vi "SH_readParams.vi"(8 "error in (no error)":errorcluster, 11 "ShapeletClass in":refnum<class "Shapelets Search Brute Force.lvclass">) -> (0 "error out":errorcluster, 1 "FeatureVectorLength":i32, 2 "NumberOfTrials":i32, 3 "ShapeletClass out":refnum<class "Shapelets Search Brute Force.lvclass">)   [LabVIEW 2016, in "Shapelets Search (Brute Force).lvlib" / "Shapelets Search Brute Force.lvclass"]
uses:
  Shapelets Search Brute Force.lvclass
  Shapelets Search Brute Force.lvclass/Shapelets Search Brute Force.ctl
panel:
  # "This VI is a part of BCI Design library, http://www.ru-bci.org \nCopyright © 2020, Sotnikov Peter, All rights reserved. License: CC BY-NC 4.0"
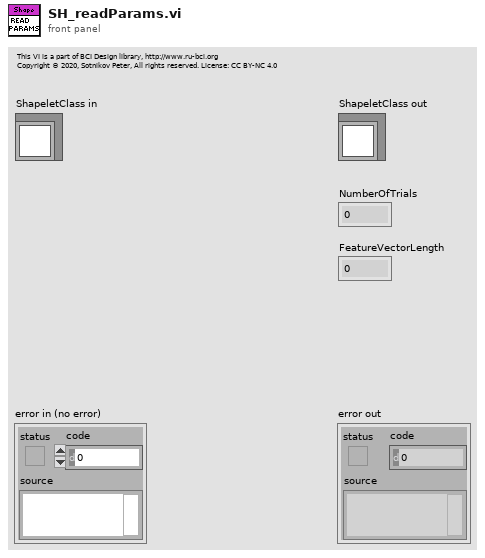
[diagram p1: front panel]
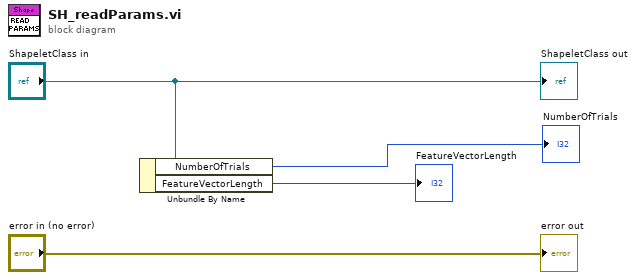
[diagram p0: block diagram]
diagram:
  n1 = Unbundle By Name("ShapeletClass in") -> ("NumberOfTrials"=→"NumberOfTrials":i32, "FeatureVectorLength"=→"FeatureVectorLength":i32)
  "error out" <- "error in (no error)"
  "ShapeletClass out" <- "ShapeletClass in"
